vi "Login.vi"(8 "error in (no error)":errorcluster, 11 "Session in":refnum<class "Session.lvclass">) -> (0 "error out":errorcluster, 3 "Session out":refnum<class "Session.lvclass">)   [LabVIEW 2016, in "Session.lvclass"]
uses:
  Session.lvclass
  Session.lvclass/Session.ctl
  Authentication/Authentication.lvclass
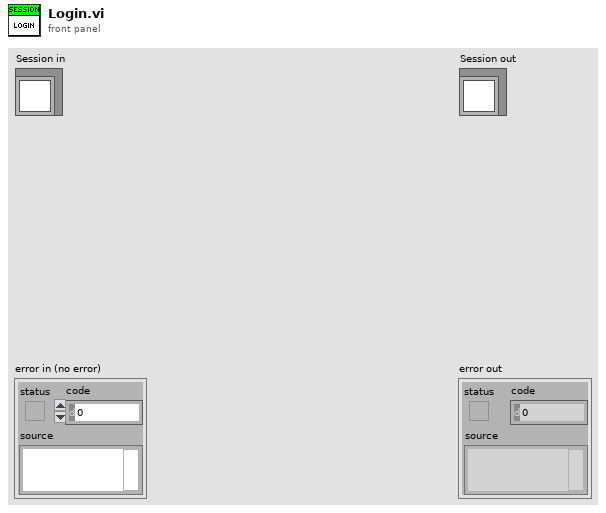
[diagram p1: front panel]
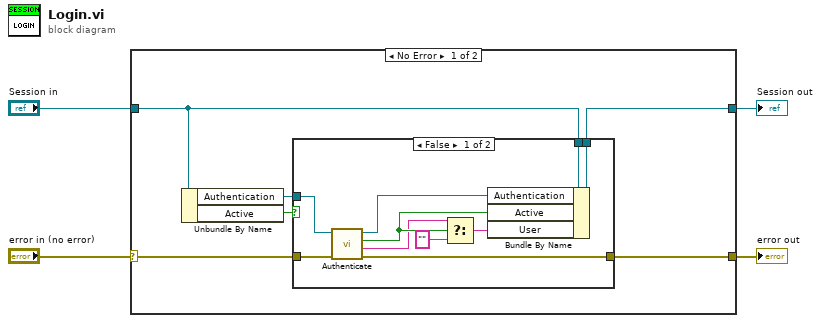
[diagram p0: block diagram]
diagram:
  n1 = case shown="No Error" "error in (no error)" {
    selector: "error in (no error)" -> [w8 w24]
    tunnel: [w7 w24] -> w3
    tunnel: [w5 w23] -> w1
    tunnel: "Session in" -> [w10 w23]
    frame No Error {
      n2 = Unbundle By Name(w10) -> ("Authentication"=w9:refnum<class "Authentication.lvclass">, "Active"=w6:bool)
      n3 = case shown="False" w6 {
        tunnel: w10 -> [w20 w22]
        tunnel: w9 -> [w19 _]
        tunnel: w8 -> [w18 w21]
        tunnel: [w17 w21] -> w7
        tunnel: [w16 w22] -> w5
        frame False {
          n4 = call "Authenticate.vi"("error in (no error)"=w18, "Authentication in"=w19) -> ("error out"=w17:errorcluster, "User"=w13:string, "Authenticated?"=w14:bool, "Authentication out"=w15:refnum<class "Authentication.lvclass">)  [unwired: 6 in]
          n5 = Select(t=w13, s=w14, f="") -> (s? t:f=w11:string)
          n6 = Bundle By Name(cluster=w20, "Authentication"=w15, "Active"=w14, "User"=w11) -> (w16:refnum<class "Session.lvclass">)
        }
        frame True {
        }
      }
    }
    frame Error {
    }
  }
  "error out" <- w3
  "Session out" <- w1
